vi "test1-ListSubModulesInDifferentSenarios.vi"(8 "error in (no error)":errorcluster, 11 "TestCase in":refnum<class "testcase-CSMSubModule.lvclass">) -> (0 "error out":errorcluster, 3 "TestCase out":refnum<class "testcase-CSMSubModule.lvclass">)   [LabVIEW 2017, in "testcase-CSMSubModule.lvclass"]
uses:
  testcase-CSMSubModule.lvclass
  <vilib>/addons/_JKI Toolkits/VI Tester/TestCase.llb/TestCase.lvclass
  src/user.lib/_NEVSTOP/Communicable State Machine(CSM)/Communicable State Machine.lvlib
  C:/Program Files (x86)/National Instruments/LabVIEW 2017/vi.lib/addons/_JKI Toolkits/VI Tester/TestCase.llb/TestCase.lvclass
panel:
  out "Error Out":errorcluster
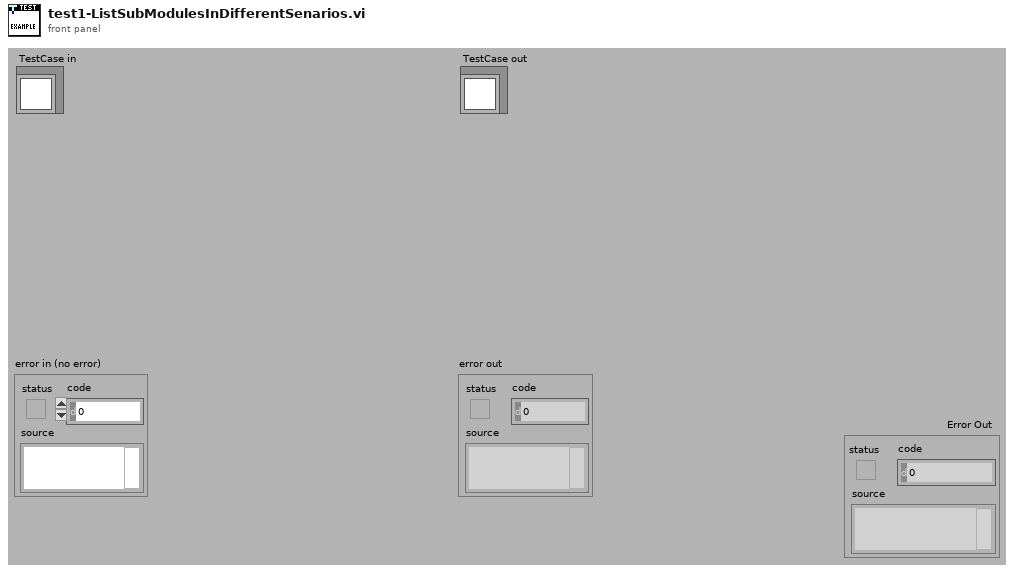
[diagram p1: front panel]
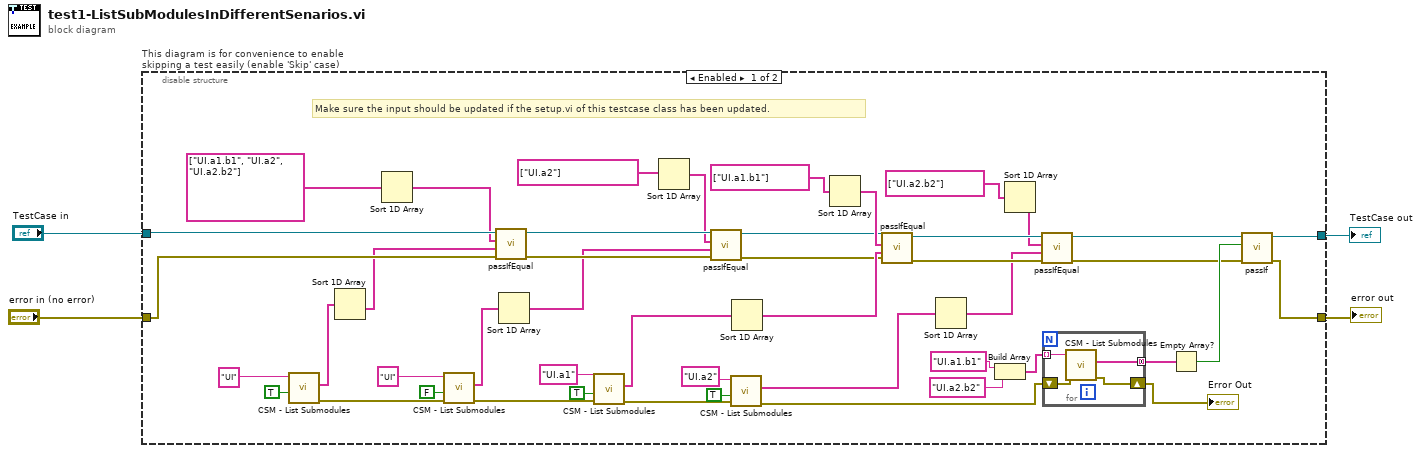
[diagram p0: block diagram]
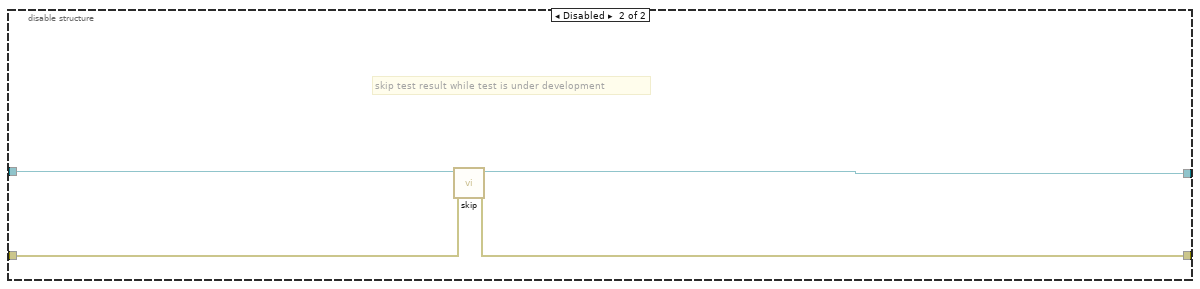
[diagram p2: hidden frame]
diagram:
  n1 = disable-structure "This diagram is for convenience to enable skipping a test easily (enable 'Skip' case)" shown="Enabled" {
    disable-tunnel: "TestCase in" -> [w48 w58]
    disable-tunnel: [w7 w56] -> w1
    disable-tunnel: [w6 w57] -> w3
    disable-tunnel: "error in (no error)" -> [w49 w55]
    frame Enabled {
      # "Make sure the input should be updated if the setup.vi of this testcase class has been updated."
      n2 = call "CSM - List Submodules.vi"("Recursive? (T)"=TRUE, "Parent Name"="UI" ("Name (\"\" to Use UUID)")) -> ("Error Out"=w46:errorcluster, "Submodules"=w50:string[])  [unwired: 7 in, 1 out]
      n3 = Sort 1D Array(array=w50) -> (sorted array=w34:string[])
      n4 = Sort 1D Array(array=string[] ["UI.a1.b1", "UI.a2", "UI.a2.b2"] ("UI's Submodules 2")) -> (sorted array=w35:string[])
      n5 = call "CSM - List Submodules.vi"("Error In"=w46, "Recursive? (T)"=FALSE, "Parent Name"="UI" ("Name (\"\" to Use UUID)")) -> ("Error Out"=w44:errorcluster, "Submodules"=w33:string[])  [unwired: 6 in, 1 out]
      n6 = call-dynamic "passIfEqual.vi"("error in (no error)"=w49, "y"=w34, "x"=w35, "TestCase in"=w48) -> ("error out"=w31:errorcluster, "TestCase out"=w32:refnum<class "testcase-CSMSubModule.lvclass">)  [unwired: 6 in]
      n7 = Sort 1D Array(array=w33) -> (sorted array=w30:string[])
      n8 = call "CSM - List Submodules.vi"("Error In"=w44, "Recursive? (T)"=TRUE, "Parent Name"="UI.a1" ("Name (\"\" to Use UUID)")) -> ("Error Out"=w42:errorcluster, "Submodules"=w25:string[])  [unwired: 6 in, 1 out]
      n9 = Sort 1D Array(array=string[] ["UI.a2"] ("UI's Submodules 2")) -> (sorted array=w28:string[])
      n10 = call-dynamic "passIfEqual.vi"("error in (no error)"=w31, "y"=w30, "x"=w28, "TestCase in"=w32) -> ("error out"=w22:errorcluster, "TestCase out"=w23:refnum<class "testcase-CSMSubModule.lvclass">)  [unwired: 6 in]
      n11 = call "CSM - List Submodules.vi"("Error In"=w42, "Recursive? (T)"=TRUE, "Parent Name"="UI.a2" ("Name (\"\" to Use UUID)")) -> ("Error Out"=w12:errorcluster, "Submodules"=w19:string[])  [unwired: 6 in, 1 out]
      n12 = Sort 1D Array(array=w25) -> (sorted array=w24:string[])
      n13 = Sort 1D Array(array=string[] ["UI.a1.b1"] ("UI's Submodules 2")) -> (sorted array=w27:string[])
      n14 = call-dynamic "passIfEqual.vi"("error in (no error)"=w22, "y"=w24, "x"=w27, "TestCase in"=w23) -> ("error out"=w20:errorcluster, "TestCase out"=w21:refnum<class "testcase-CSMSubModule.lvclass">)  [unwired: 6 in]
      n15 = Sort 1D Array(array=w19) -> (sorted array=w18:string[])
      n16 = Build Array("UI.a1.b1" ("Name (\"\" to Use UUID)"), "UI.a2.b2" ("Name (\"\" to Use UUID)")) -> (w13:string[])
      n17 = Sort 1D Array(array=string[] ["UI.a2.b2"] ("UI's Submodules 2")) -> (sorted array=w16:string[])
      n18 = call-dynamic "passIfEqual.vi"("error in (no error)"=w20, "y"=w18, "x"=w16, "TestCase in"=w21) -> ("error out"=w8:errorcluster, "TestCase out"=w9:refnum<class "testcase-CSMSubModule.lvclass">)  [unwired: 6 in]
      n19 = for {
        tunnel: w13 -> [w54] mode=indexing
        shift-right: [w52] -> w5
        shift-left: w12 -> [w53]
        tunnel: [w51] -> w11 mode=concatenating
        n20 = call "CSM - List Submodules.vi"("Error In"=w53, "Parent Name"=w54) -> ("Error Out"=w52:errorcluster, "Submodules"=w51:string[])  [unwired: 7 in, 1 out]
      }
      "Error Out" <- w5
      n21 = Empty Array?(array=w11) -> (empty?=w10:bool)
      n22 = call-dynamic "passIf.vi"("error in (no error)"=w8, "pass"=w10, "TestCase in"=w9) -> ("error out"=w6:errorcluster, "TestCase out"=w7:refnum<class "testcase-CSMSubModule.lvclass">)  [unwired: 7 in]
    }
    frame Disabled {
      # "skip test result while test is under development"
      n23 = call <vilib>:"skip.vi"("error in (no error)"=w55, "TestCase in"=w58) -> ("error out"=w57:errorcluster, "TestCase out"=w56:refnum<class "testcase-CSMSubModule.lvclass">)  [unwired: 8 in]
    }
  }
  "error out" <- w3
  "TestCase out" <- w1
